vi "TCP_writeread.vi"(9 "写入数据":u32 format="%02x") -> ()   [LabVIEW 2012]
uses:
  S7Ref.vi
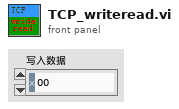
[diagram p1: front panel]
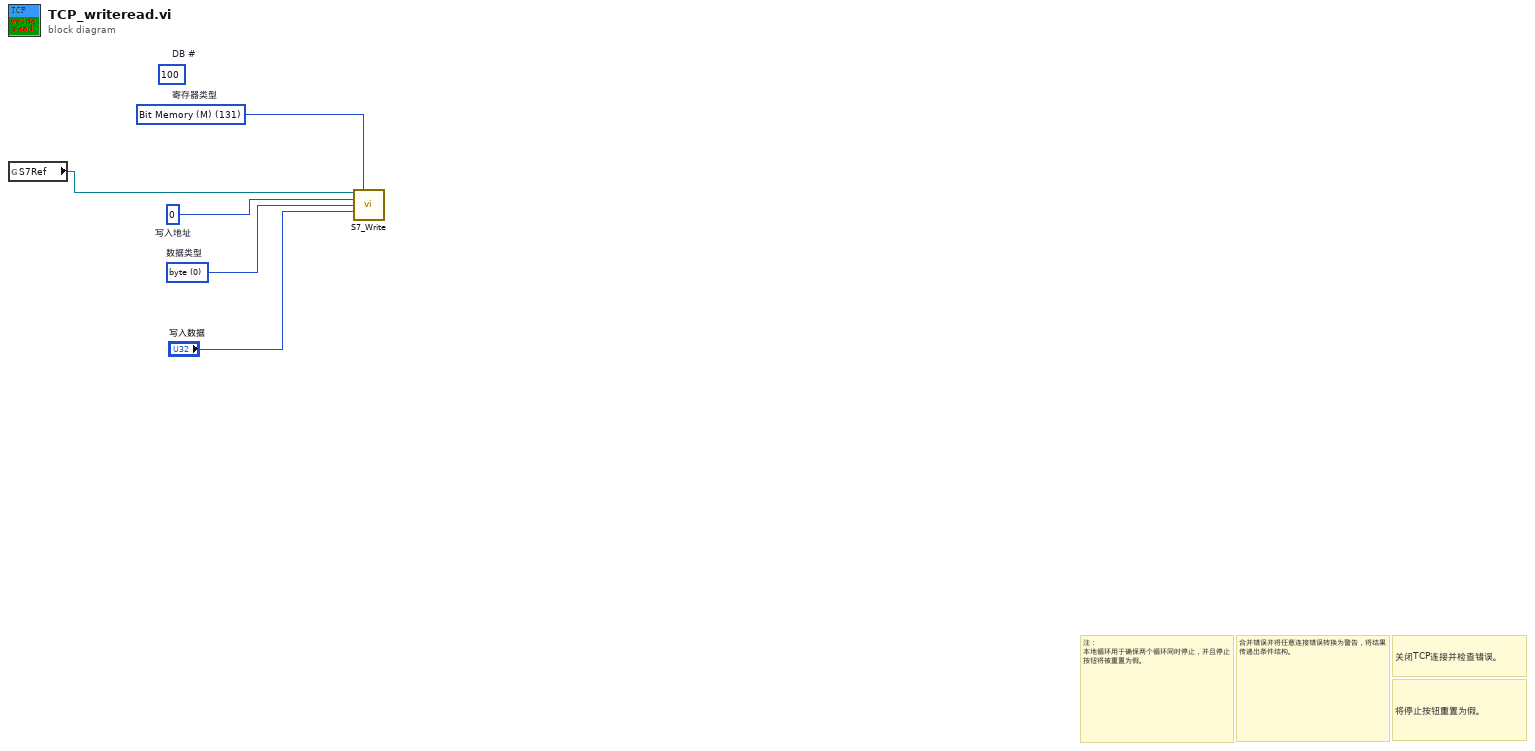
[diagram p0: block diagram]
diagram:
  w4 = u16 0 items=["byte", "word", "Dword"]  # 数据类型
  w3 = u32 0  # 写入地址
  (unwired) u16 100  # DB #
  w5 = u8 131 items=["I/O (P)"=128, "Input (I)"=129, "Output (Q)"=130, "Bit Memory (M)"=131, "Data (DB)"=132, "Instance Data (DI)"=133, "Local Data (L)"=134, "Predecessor Local Data (VL)"=135]  # 寄存器类型
  # "将停止按钮重置为假。"
  # "关闭TCP连接并检查错误。"
  # "合并错误并将任意连接错误转换为警告，将结果传递出条件结构。"
  # "注： 本地循环用于确保两个循环同时停止，并且停止按钮将被重置为假。"
  n1 = global read "S7Ref.vi" "S7Ref"() -> (w1:refnum<k5>)
  n2 = call "S7_Write.vi"("TCP"=w1, "寄存器类型"=w5, "写入地址"=w3, "数据类型"=w4, "写入数据"="写入数据") -> ()  [unwired: 8 in, 3 out]
